vi "FINAL.vi"() -> ()   [LabVIEW 2019]
doc: "This example demonstrates how to continuously acquire buffered voltage measurements using a DAQmx device. It uses software events to ensure that the program does not become unresponsive while waiting for samples to become available.\n\nFor instructions on how to connect your signals to the DAQ device, refer to your device documentation."
uses:
  <vilib>/Utility/error.llb/DialogType.ctl
  <vilib>/DAQmx/read.llb/DAQmx Read (Analog 1D Wfm NChan NSamp).vi
  <vilib>/DAQmx/create/channels.llb/DAQmx Create Channel (AI-Voltage-Basic).vi
  <vilib>/DAQmx/configure/timing.llb/DAQmx Timing (Sample Clock).vi
  <vilib>/DAQmx/configure/task.llb/DAQmx Configure Logging (TDMS).vi
  <vilib>/DAQmx/configure/trigger.llb/DAQmx Start Trigger (Analog Window).vi
  <vilib>/DAQmx/miscellaneous.llb/DAQmx Fill In Error Info.vi
  <resource>/objmgr/daqmx.rc
panel:
  in  "stop":bool
  out "TDMS file path":path
  out "# of Channels":dbl
  out "Samples/event loop":dbl
  out "Channel Config":dbl
  out "Min Voltage":dbl
  out "Max Voltage":dbl
  in  "Stop":bool
  out "Waveform Graph":waveform(dbl)[](graph)
  out "Actual Sample Rate":dbl format="%0.2f"
  # "Channel Settings"
  # "Acquired Data"
  # "Timing Settings"
  # "Trigger Settings"
  # "Logging Settings"
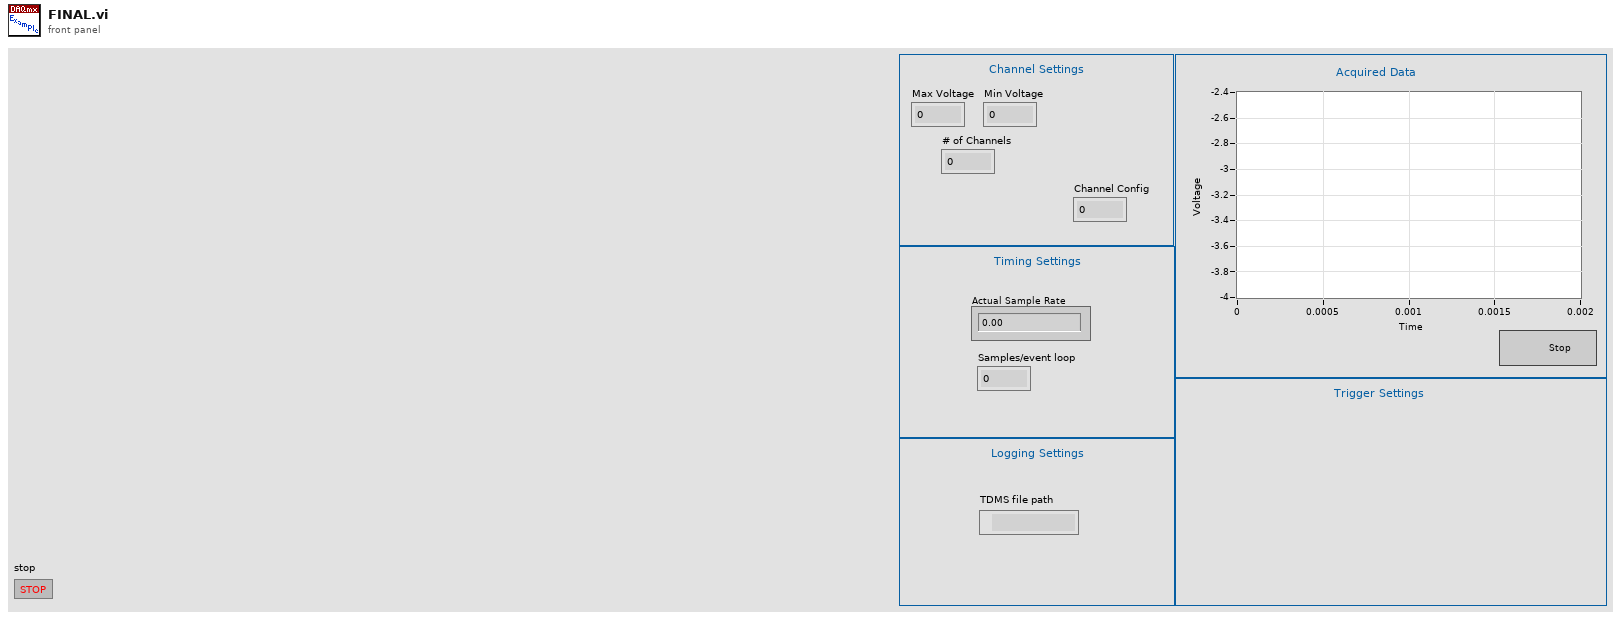
[diagram p1: front panel]
types:
  T1 = typedef "DialogType.ctl" = u16
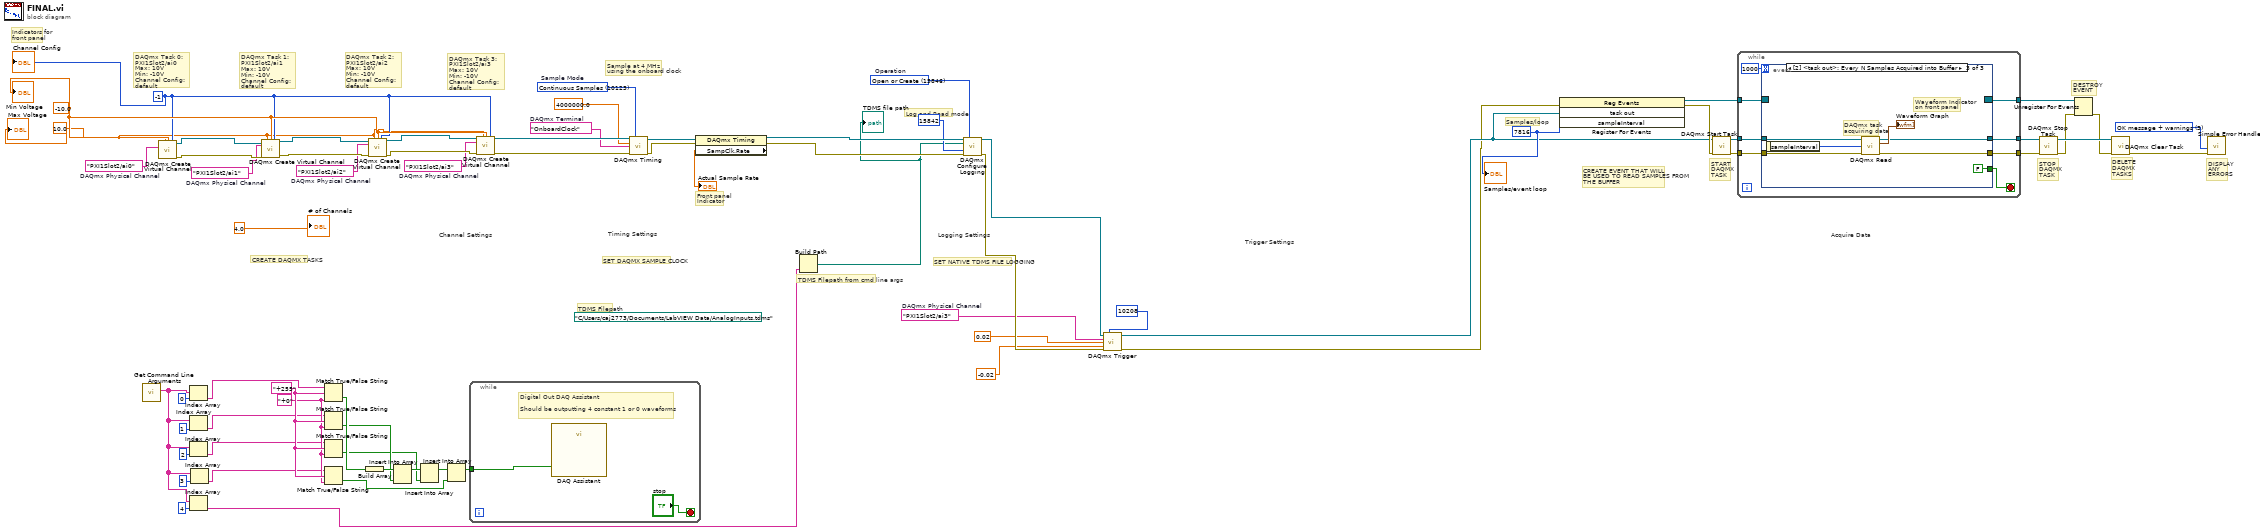
[diagram p0: block diagram]
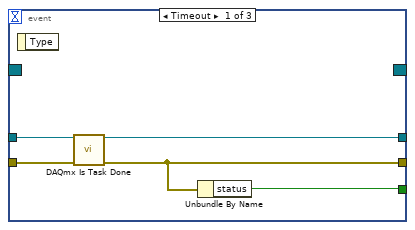
[diagram p2: hidden frame]
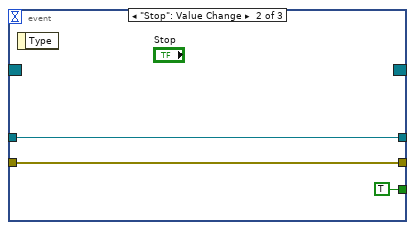
[diagram p3: hidden frame]
diagram:
  w14 = "+0"
  w15 = "+255"
  w24 = tag "PXI1Slot2/ai3"  # DAQmx Physical Channel
  w34 = -1
  w33 = 7816
  (unwired) path "C:/Users/caj2773/Documents/LabVIEW Data/AnalogInputs.tdms"
  w42 = tag "OnboardClock"  # DAQmx Terminal
  w38 = tag "PXI1Slot2/ai3"  # DAQmx Physical Channel
  w39 = tag "PXI1Slot2/ai2"  # DAQmx Physical Channel
  w40 = tag "PXI1Slot2/ai1"  # DAQmx Physical Channel
  w41 = tag "PXI1Slot2/ai0"  # DAQmx Physical Channel
  w35 = -10.0
  w1 = 10.0
  w52 = T1 3 items=["no dialog", "OK message", "continue or stop message", "OK message + warnings", "continue/stop + warnings"] ("type of dialog (OK msg:1)")
  w62 = 15846 items=["Open"=10437, "Open or Create"=15846, "Create or Replace"=15847, "Create"=15848]  # Operation
  w67 = 10123 items=["Finite Samples"=10178, "Continuous Samples"=10123, "Hardware Timed Single Point"=12522]  # Sample Mode
  # "TDMS Filepath from cmd line args"
  # "DISPLAY\nANY\nERRORS"
  # "DELETE\nDAQMX\nTASKS"
  # "DESTROY\nEVENT"
  # "STOP\nDAQMX\nTASK"
  # "START\nDAQMX\nTASK"
  # "Samples/loop"
  # "CREATE EVENT THAT WILL\nBE USED TO READ SAMPLES FROM\nTHE BUFFER"
  # "Sample at 4 MHz\nusing the onboard clock"
  # "SET NATIVE TDMS FILE LOGGING"
  # "SET DAQMX SAMPLE CLOCK"
  # "Front panel\nIndicator"
  # "TDMS Filepath"
  # "Log and Read mode"
  # "DAQmx Task 3:\nPXI1Slot2/ai3\nMax: 10V\nMin: -10V\nChannel Config: default"
  # "Indicators for\nfront panel"
  # "DAQmx Task 2:\nPXI1Slot2/ai2\nMax: 10V\nMin: -10V\nChannel Config: default"
  # "DAQmx Task 1:\nPXI1Slot2/ai1\nMax: 10V\nMin: -10V\nChannel Config: default"
  # "DAQmx Task 0:\nPXI1Slot2/ai0\nMax: 10V\nMin: -10V\nChannel Config: default"
  # "CREATE DAQMX TASKS"
  # "Trigger Settings"
  # "Acquire Data"
  # "Logging Settings"
  # "Timing Settings"
  # "Channel Settings"
  n1 = call <vilib>:"Get Command Line Arguments.vi"() -> ("arguments"=w5:string[])  [unwired: 9 in, 2 out]
  n2 = call-poly <vilib>:"DAQmx Create Virtual Channel.vi"("maximum value"=w1, "minimum value"=w35, "input terminal configuration"=w34, "physical channels"=w41) -> ("task out"=w48:refnum<k21>, "error out"=w45:errorcluster)  [unwired: 10 in]
  n3 = Index Array(array=w5, index=0) -> (element=w9:string)
  n4 = Index Array(array=w5, index=1) -> (element=w8:string)
  n5 = Index Array(array=w5, index=2) -> (element=w7:string)
  n6 = Index Array(array=w5, index=4) -> (element=w3:string)
  n7 = Index Array(array=w5, index=3) -> (element=w6:string)
  n8 = call-poly <vilib>:"DAQmx Create Virtual Channel.vi"("task in"=w48, "maximum value"=w1, "minimum value"=w35, "input terminal configuration"=w34, "physical channels"=w40, "error in"=w45) -> ("task out"=w47:refnum<k21>, "error out"=w44:errorcluster)  [unwired: 8 in]
  n9 = Match True/False String(2:w14, 3:w15, 4:w8) -> (0:w18:bool)  [unwired: 1 out]
  n10 = Match True/False String(2:w14, 3:w15, 4:w7) -> (0:w17:bool)  [unwired: 1 out]
  n11 = Match True/False String(2:w14, 3:w15, 4:w6) -> (0:w16:bool)  [unwired: 1 out]
  n12 = Match True/False String(2:w14, 3:w15, 4:w9) -> (0:w19:bool)  [unwired: 1 out]
  n13 = Build Array(w19) -> (w23:bool[])
  n14 = call-poly <vilib>:"DAQmx Create Virtual Channel.vi"("task in"=w47, "maximum value"=w1, "minimum value"=w35, "input terminal configuration"=w34, "physical channels"=w39, "error in"=w44) -> ("task out"=w46:refnum<k21>, "error out"=w43:errorcluster)  [unwired: 8 in]
  n15 = Insert Into Array(array=w23, new element=w18) -> (w20:bool[])  [unwired: 1 in]
  n16 = Insert Into Array(array=w20, new element=w17) -> (w21:bool[])  [unwired: 1 in]
  n17 = Insert Into Array(array=w21, new element=w16) -> (w22:bool[])  [unwired: 1 in]
  n18 = while {
    tunnel: w22 -> [w71]
    stop <- "stop" stop-if-true
    # "Digital Out DAQ Assistant\n\nShould be outputting 4 constant 1 or 0 waveforms"
    n19 = call "DAQ Assistant"("data"=w71) -> ()  [unwired: 17 in, 2 out]
  }
  n20 = call-poly <vilib>:"DAQmx Create Virtual Channel.vi"("task in"=w46, "maximum value"=w1, "minimum value"=w35, "input terminal configuration"=w34, "physical channels"=w38, "error in"=w43) -> ("task out"=w65:refnum<k21>, "error out"=w66:errorcluster)  [unwired: 8 in]
  n21 = call-poly <vilib>:"DAQmx Timing.vi"("task/channels in"=w65, "sample mode"=w67, "rate"=4000000.0, "source"=w42, "error in"=w66) -> ("task out"=w69:refnum<k21>, "error out"=w68:errorcluster)  [unwired: 9 in]
  n22 = property class="DAQmx Timing"(reference=w69, error in=w68) -> (reference out=w64:refnum<k21>, error out=w63:errorcluster, "SampClk.Rate"=→"Actual Sample Rate":dbl)
  n23 = Build Path(name or relative path=w3) -> (appended path=w2:path)  [unwired: 1 in]
  "TDMS file path" <- w2
  n24 = call-poly <vilib>:"DAQmx Configure Logging.vi"("task/channels in"=w64, "operation"=w62, "file path"=w2, "logging mode"=15842, "error in"=w63) -> ("task out"=w29:refnum<k21>, "error out"=w28:errorcluster)  [unwired: 9 in]
  n25 = call-poly <vilib>:"DAQmx Trigger.vi"("task/channels in"=w29, "when"=10208, "source"=w24, "window top"=0.02, "window bottom"=-0.02, "error in"=w28) -> ("task out"=w31:refnum<k21>, "error out"=w30:errorcluster)  [unwired: 8 in]
  n26 = register-events(error in=w30, w31, w33) -> (reference out=w59:refnum<event-registration>, error out=w58:errorcluster)  [unwired: 1 in]
  n27 = call <vilib>:"DAQmx Start Task.vi"("task/channels in"=w31, "error in"=w58) -> ("task out"=w56:refnum<k21>, "error out"=w57:errorcluster)  [unwired: 12 in]
  n28 = while {
    tunnel: w59 -> [w79]
    tunnel: w57 -> [w78]
    tunnel: w56 -> [w77]
    tunnel: [w76] -> w53
    tunnel: [w75] -> w55
    tunnel: [w74] -> w51
    stop <- w73 stop-if-true
    n29 = event shown="[2] <task out>: Every N Samples Acquired into Buffer" {
      selector: w79 -> [_ _ _]
      dyn-events: [_ _ _] -> w75
      timeout: 1000 ("Event Timeout") -> [_ _ _]
      tunnel: w78 -> [w83 w86 w92]
      tunnel: w77 -> [w84 w87 w93]
      tunnel: [w82 w87 w90] -> w76
      tunnel: [w81 w86 w89] -> w74
      tunnel: [w80 TRUE FALSE] -> w73
      event Timeout {
        n30 = event-data() -> ()  [unwired: 1 in, 1 out]
        n31 = call <vilib>:"DAQmx Is Task Done.vi"("task/channels in"=w84, "error in"=w83) -> ("task out"=w82:refnum<k21>, "error out"=w81:errorcluster)  [unwired: 11 in, 1 out]
        n32 = Unbundle By Name(w81) -> ("status"=w80:bool)
      }
      event "Stop": Value Change {
        n33 = event-data() -> ()  [unwired: 1 in, 1 out]
      }
      event Every N Samples Acquired into Buffer {
        # "Waveform Indicator\non front panel"
        # "DAQmx task\nacquiring data"
        n34 = event-data() -> ("sampleInterval"=w91:u32)  [unwired: 1 in]
        n35 = call-poly <vilib>:"DAQmx Read.vi"("task/channels in"=w93, "number of samples per channel"=w91, "error in"=w92) -> ("task out"=w90:refnum<k21>, "data"=→"Waveform Graph":waveform(dbl)[], "error out"=w89:errorcluster)  [unwired: 10 in]
      }
    }
  }
  n36 = call <vilib>:"DAQmx Stop Task.vi"("task/channels in"=w53, "error in"=w51) -> ("task out"=w54:refnum<k21>, "error out"=w50:errorcluster)  [unwired: 12 in]
  n37 = Unregister For Events(event registration refnum=w55, error in=w50) -> (error out=w49:errorcluster)
  n38 = call <vilib>:"DAQmx Clear Task.vi"("task in"=w54, "error in"=w49) -> ("error out"=w61:errorcluster)  [unwired: 13 in]
  n39 = call <vilib>:"Simple Error Handler.vi"("type of dialog (OK msg:1)"=w52, "error in (no error)"=w61) -> ()  [unwired: 3 in, 5 out]
  "Max Voltage" <- w1
  "Min Voltage" <- w35
  "Channel Config" <- w34
  "Samples/event loop" <- w33
  "# of Channels" <- 4.0
